vi "V7310.Angle.Set.vi"(6 "timeout ms (5000)":i32=5000, 8 "error in":errorcluster, 10 "Angle":dbl format="%.1f", 11 "Connection in":refnum<k5>) -> (0 "error out":errorcluster, 3 "Connection out":refnum<k5>)   [LabVIEW 2016]
uses:
  LowLevel/V7310.Commands.ctl
panel:
  out "Data out":string
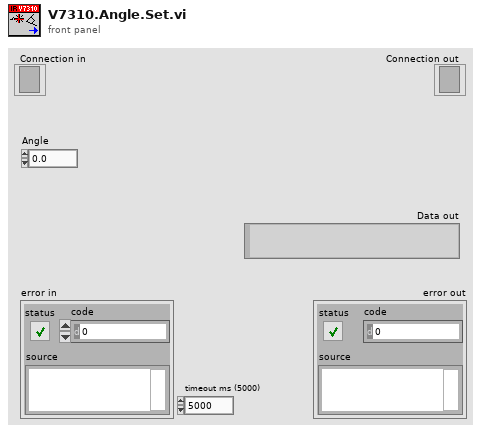
[diagram p1: front panel]
types:
  T1 = typedef "V7310.Commands.ctl" = enum16{"Start", "Stop", "GetStatus", "GetVarNames", "GetJobNames", "SetJob", "GetJob", "SetVars", "GetVars", "SetLayoutPosition", "SetRotation", "GetMessageID", "GetMessages", "ConfirmMessages", "DeleteMessages", "SetRTC", "GetRTC", "SetVarPosition", "SetIntensity", "GetIntensity", "SetStartTriggerDelay", "GetStartTriggerDelay", "SetStopTriggerDelay", "GetStopTriggerDelay", "SetConsecutiveTriggerDelay", "GetConsecutiveTriggerDelay", "SetMarkSpeed", "GetMarkSpeed"}
  T2 = typedef "V7310.ErrorLevels.ctl" = enum16{"OK", "Warning", "Error"}
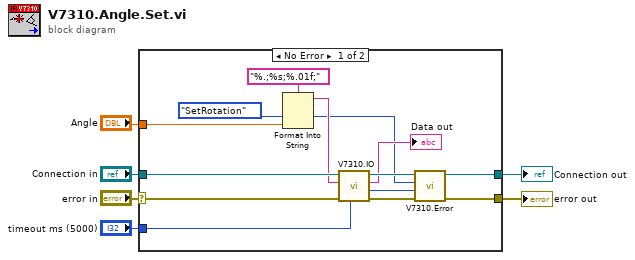
[diagram p0: block diagram]
diagram:
  n1 = case shown="No Error" "error in" {
    selector: "error in" -> [w16 w19]
    tunnel: "Connection in" -> [w17 w20]
    tunnel: [w18 w20] -> w5
    tunnel: "timeout ms (5000)" -> [w15 _]
    tunnel: [w10 w19] -> w2
    tunnel: "Angle" -> [w7 _]
    frame No Error {
      w8 = V7310.Commands."SetRotation" ("Cmd")
      n2 = Format Into String(format string="%.;%s;%.01f;", w8, w7) -> (resulting string=w13:string)  [unwired: 2 in, 1 out]
      n3 = call "V7310.IO.vi"("timeout ms (5000)"=w15, "error in"=w16, "Data in"=w13, "Connection in"=w17) -> ("error out"=w11:errorcluster, "Error Level"=w12:T2, "Data out"=→"Data out":string, "Connection out"=w18:refnum<k5>)  [unwired: 4 in]
      n4 = call "V7310.Error.vi"("error in"=w11, "Error Level"=w12, "Cmd"=w8) -> ("error out"=w10:errorcluster)  [unwired: 8 in]
    }
    frame Error {
    }
  }
  "Connection out" <- w5
  "error out" <- w2
